vi "PXI-4132 Initialization - Add DCPower Channel.vi"(8 "error in (no error)":errorcluster, 9 "Channel #":i32, 10 "Channel Name":string, 11 "Device Item Ref In":T1 format="%.0x") -> (0 "error out":errorcluster, 3 "Device Item Ref Out":T1 format="%.0x")   [LabVIEW 2013, in "PXI-4132 Custom Device.lvlib"]
uses:
  PXI-4132 Custom Device.lvlib
  <vilib>/NI Veristand/Custom Device API/Custom Device Item Ref.ctl
  <vilib>/NI Veristand/Custom Device API/Custom Device Channel Type.ctl
  <vilib>/NI Veristand/Custom Device API/Custom Device Channel.ctl
  Channel Type.ctl
  Channel Sense.ctl
  <vilib>/NI Veristand/Custom Device API/Set Item Property (I32).vi
  PXI-4132 Global Variable.vi
  <vilib>/NI VeriStand/Custom Device API/Custom Device API.lvlib
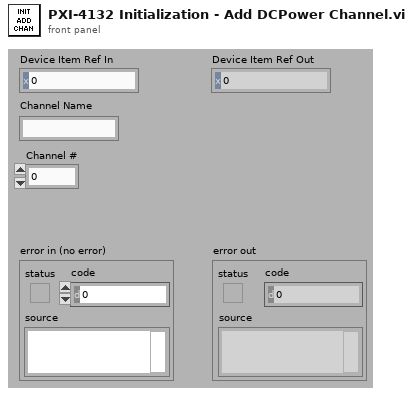
[diagram p1: front panel]
types:
  T1 = typedef "Custom Device API.lvlib/Custom Device Item Ref.ctl" = u64
  T2 = typedef "PXI-4132 Custom Device.lvlib/Channel Sense.ctl" = i32
  T3 = typedef "PXI-4132 Custom Device.lvlib/Channel Type.ctl" = i32
  T4 = typedef "Custom Device API.lvlib/Custom Device Channel Type.ctl" = enum16{"Input", "Output"}
  T5 = typedef "Custom Device API.lvlib/Custom Device Channel.ctl" = cluster{"Type":T4, "Units":string, "Default Value":dbl, "Faultable":bool, "Scalable":bool}
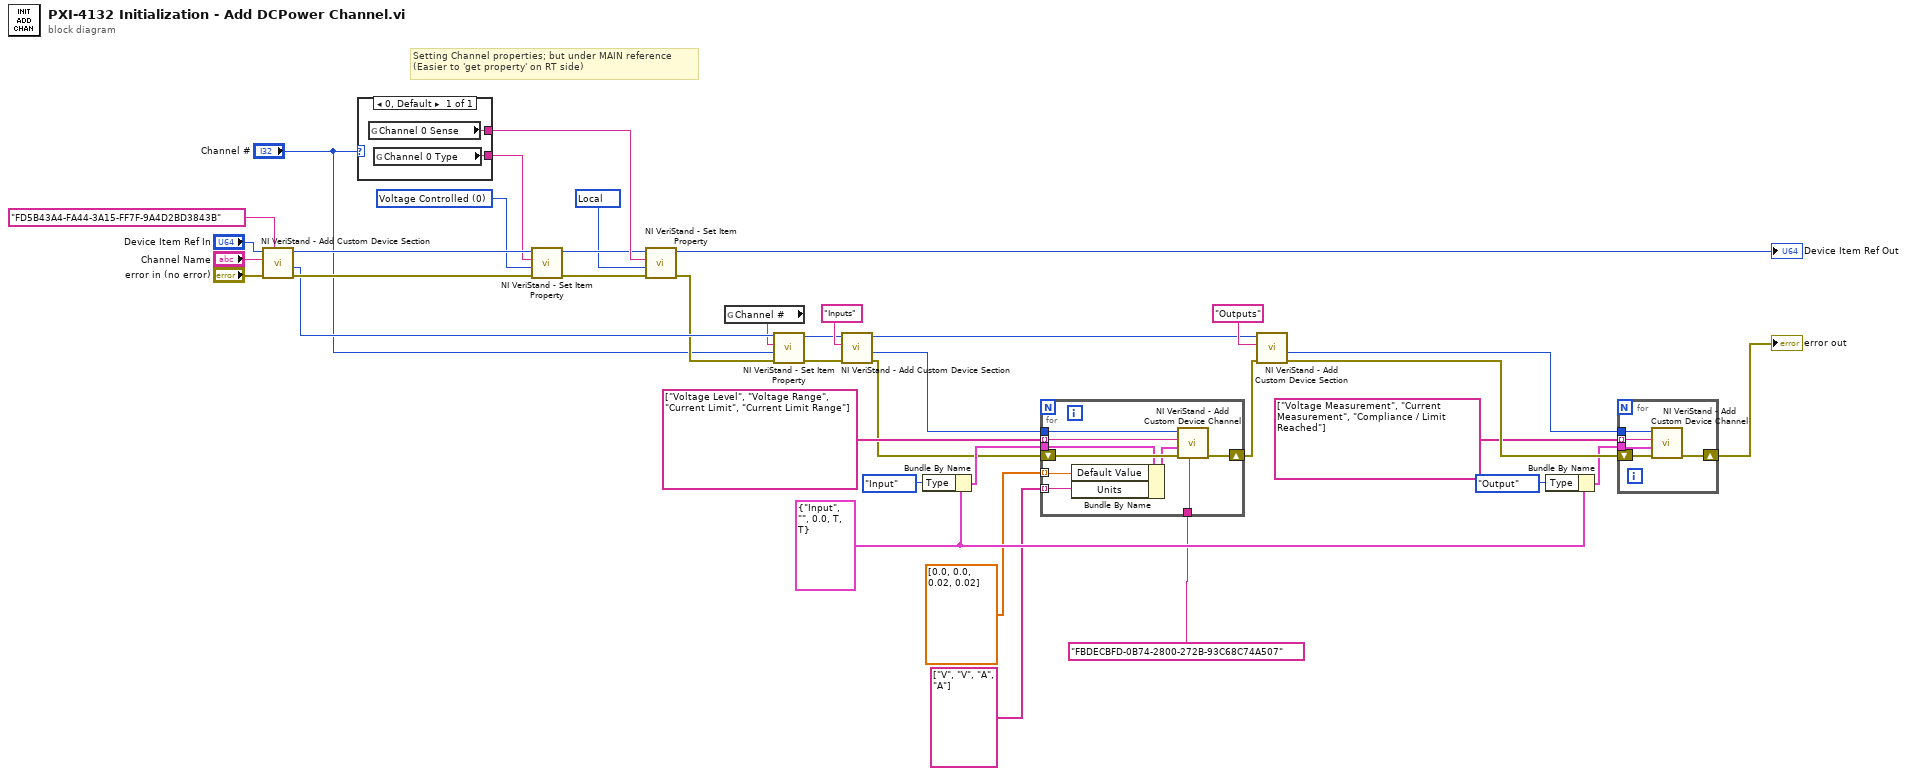
[diagram p0: block diagram]
diagram:
  w4 = T2 1008 items=["Local"=1008, "Remote"=1009] ("Channel Sense")
  w15 = T3 0 items=["Voltage Controlled", "Current Controlled"] ("Channel Type")
  w22 = T5 {"Type"=enum."Input", "Units"="", "Default Value"=0.0, "Faultable"=TRUE, "Scalable"=TRUE} ("Channel")
  # "Setting Channel properties; but under MAIN reference\n(Easier to 'get property' on RT side)"
  n1 = call <vilib>:"NI VeriStand - Add Custom Device Section.vi"("GUID (Default Section)"="FD5B43A4-FA44-3A15-FF7F-9A4D2BD3843B", "error in (no error)"="error in (no error)", "Section Name"="Channel Name", "Parent Ref in"="Device Item Ref In") -> ("error out"=w16:errorcluster, "Section Ptr"=w9:T1, "Parent Ref out"=w20:T1)  [unwired: 4 in, 1 out]
  n2 = case shown="0, Default" "Channel #" {
    tunnel: [w39] -> w19
    tunnel: [w38] -> w14
    frame 0, Default {
      n3 = global read "PXI-4132 Global Variable.vi" "Channel 0 Sense"() -> (w38:string)
      n4 = global read "PXI-4132 Global Variable.vi" "Channel 0 Type"() -> (w39:string)
    }
  }
  n5 = call-poly <vilib>:"NI VeriStand - Set Item Property.vi"("error in (no error)"=w16, "Value"=w15, "Property Name"=w19, "Item Ref in"=w20) -> ("error out"=w8:errorcluster, "Item Ref out"=w13:T1)  [unwired: 5 in, 1 out]
  n6 = call-poly <vilib>:"NI VeriStand - Set Item Property.vi"("Value"=w4, "Property Name"=w14, "Item Ref in"=w13) -> ("Item Ref out"=→"Device Item Ref Out":T1)  [unwired: 6 in, 2 out]
  n7 = global read "PXI-4132 Global Variable.vi" "Channel #"() -> (w6:string)
  n8 = call-poly <vilib>:"NI VeriStand - Set Item Property.vi"("error in (no error)"=w8, "Value"="Channel #", "Property Name"=w6, "Item Ref in"=w9) -> ("error out"=w7:errorcluster, "Item Ref out"=w10:T1)  [unwired: 5 in, 1 out]
  n9 = call <vilib>:"NI VeriStand - Add Custom Device Section.vi"("error in (no error)"=w7, "Section Name"="Inputs", "Parent Ref in"=w10) -> ("error out"=w33:errorcluster, "Section Ptr"=w34:T1, "Parent Ref out"=w18:T1)  [unwired: 5 in, 1 out]
  n10 = Bundle By Name(cluster=w22, "Type"=Custom_Device_Channel_Type."Input") -> (w35:T5)
  n11 = for {
    tunnel: w34 -> [w48]
    tunnel: string[] ["Voltage Level", "Voltage Range", "Current Limit", "Current Limit Range"] -> [w46] mode=indexing
    tunnel: w35 -> [w43]
    shift-right: [w45] -> w23
    shift-left: w33 -> [w47]
    tunnel: "FBDECBFD-0B74-2800-272B-93C68C74A507" ("Section Name") -> [w44]
    tunnel: dbl[] [0.0, 0.0, 0.02, 0.02] -> [w41] mode=indexing
    tunnel: string[] ["V", "V", "A", "A"] -> [w40] mode=indexing
    n12 = Bundle By Name(cluster=w43, "Default Value"=w41, "Units"=w40) -> (w42:T5)
    n13 = call <vilib>:"NI VeriStand - Add Custom Device Channel.vi"("GUID (Default Channel)"=w44, "error in (no error)"=w47, "Channel"=w42, "Channel Name"=w46, "Parent Ref in"=w48) -> ("error out"=w45:errorcluster)  [unwired: 3 in, 3 out]
  }
  n14 = call <vilib>:"NI VeriStand - Add Custom Device Section.vi"("error in (no error)"=w23, "Section Name"="Outputs", "Parent Ref in"=w18) -> ("error out"=w31:errorcluster, "Section Ptr"=w30:T1)  [unwired: 5 in, 2 out]
  n15 = Bundle By Name(cluster=w22, "Type"=Custom_Device_Channel_Type."Output") -> (w29:T5)
  n16 = for {
    tunnel: w30 -> [w53]
    tunnel: string[] ["Voltage Measurement", "Current Measurement", "Compliance / Limit Reached"] -> [w51] mode=indexing
    tunnel: w29 -> [w50]
    shift-right: [w49] -> w21
    shift-left: w31 -> [w52]
    n17 = call <vilib>:"NI VeriStand - Add Custom Device Channel.vi"("error in (no error)"=w52, "Channel"=w50, "Channel Name"=w51, "Parent Ref in"=w53) -> ("error out"=w49:errorcluster)  [unwired: 4 in, 3 out]
  }
  "error out" <- w21
